vi "OPO_TCP_Client_Read.vi"(8 "error in (no error)":errorcluster, 11 "port":u16) -> (0 "error out":errorcluster, 2 "value read":i32, 3 "TCP Network Connection out":refnum<k5>)   [LabVIEW 2020]
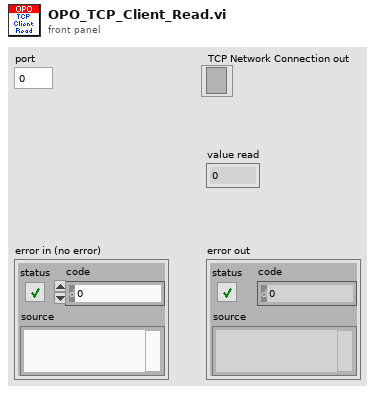
[diagram p1: front panel]
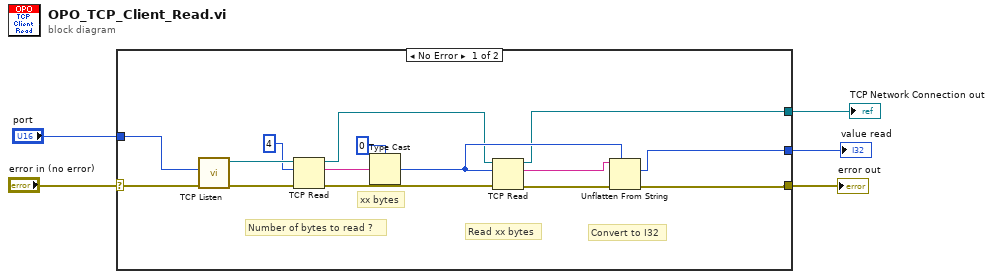
[diagram p0: block diagram]
diagram:
  n1 = case shown="No Error" "error in (no error)" {
    selector: "error in (no error)" -> [w8 w21]
    tunnel: [w19 _] -> w5
    tunnel: "port" -> [w9 _]
    tunnel: [w7 w21] -> w2
    tunnel: [w6 _] -> w1
    frame No Error {
      # "xx bytes"
      # "Convert to I32"
      # "Read xx bytes"
      # "Number of bytes to read ?"
      n2 = call <vilib>:"TCP Listen.vi"("error in (no error)"=w8, "port"=w9) -> ("error out"=w12:errorcluster, "connection ID"=w11:refnum<k5>)  [unwired: 5 in, 3 out]
      n3 = TCP Read(connection ID=w11, bytes to read=4, error in (no error)=w12) -> (connection ID out=w16:refnum<k5>, data out=w14:string, error out=w13:errorcluster)  [unwired: 2 in]
      n4 = Type Cast(type=0, x=w14) -> (*(type *) &x=w20:i32)
      n5 = TCP Read(connection ID=w16, bytes to read=w20, error in (no error)=w13) -> (connection ID out=w19:refnum<k5>, data out=w18:string, error out=w17:errorcluster)  [unwired: 2 in]
      n6 = Unflatten From String(type=w20, binary string=w18, error in (no error)=w17) -> (value=w6:i32, error out=w7:errorcluster)  [unwired: 2 in, 1 out]
    }
    frame Error {
    }
  }
  "TCP Network Connection out" <- w5
  "error out" <- w2
  "value read" <- w1
